vi "CreatUTMgrRes.vi"(8 "错误输入（无错误）":errorcluster) -> (0 "错误输出":errorcluster, 3 "返回值":i32)   [LabVIEW 2018]
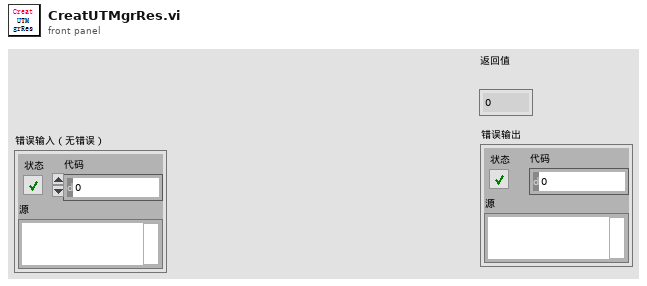
[diagram p1: front panel]
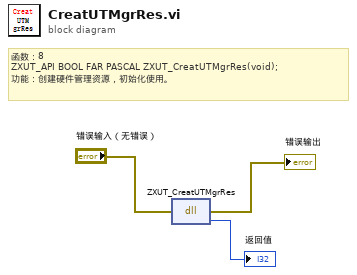
[diagram p0: block diagram]
diagram:
  # "函数：8\nZXUT_API BOOL\tFAR PASCAL ZXUT_CreatUTMgrRes(void);\n功能：创建硬件管理资源，初始化使用。"
  n1 = dll-call lib="PTH2Rabs E软件项目超声超声子VI函数VI\tTCG处理ZXUTConfigMgr.dll" fn="ZXUT_CreatUTMgrRes"(error in="错误输入（无错误）") -> (error out=→"错误输出":errorcluster, "返回值"=→"返回值":i32)  [unwired: 2 in, 1 out]
